vi "Memory.Pointer.Read All.vi"   [LabVIEW 2016]
uses:
  Memory.Pointer.lvclass
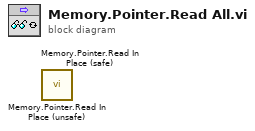
[diagram p0: block diagram]
diagram:
  n1 = call "Memory.Pointer.Read In Place (unsafe).vi"() -> ()  [unwired: 8 in, 4 out]
  n2 = call "Memory.Pointer.Read In Place (safe).vi"() -> ()  [unwired: 8 in, 4 out]
